vi "read_data.vi"(8 "error in (no error)":errorcluster, 10 "bytes to read":i32, 11 "MH100301DMC in":refnum<class "StageMH100301DMC.lvclass">) -> (0 "error out":errorcluster, 2 "hex data string":string, 3 "MH100301DMC out":refnum<class "StageMH100301DMC.lvclass">)   [LabVIEW 2010]
uses:
  StageMH100301DMC.lvclass
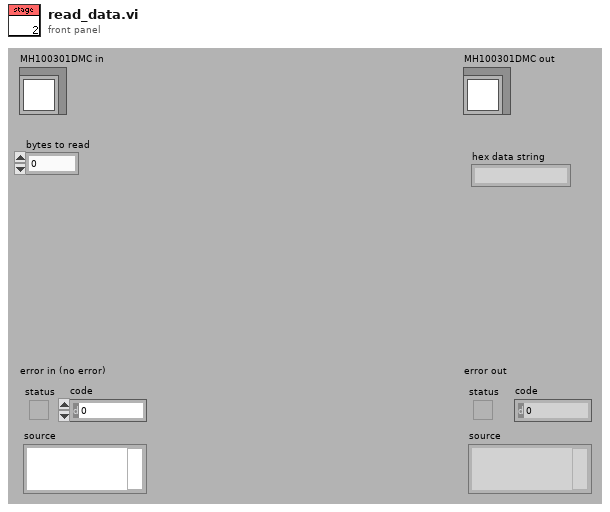
[diagram p1: front panel]
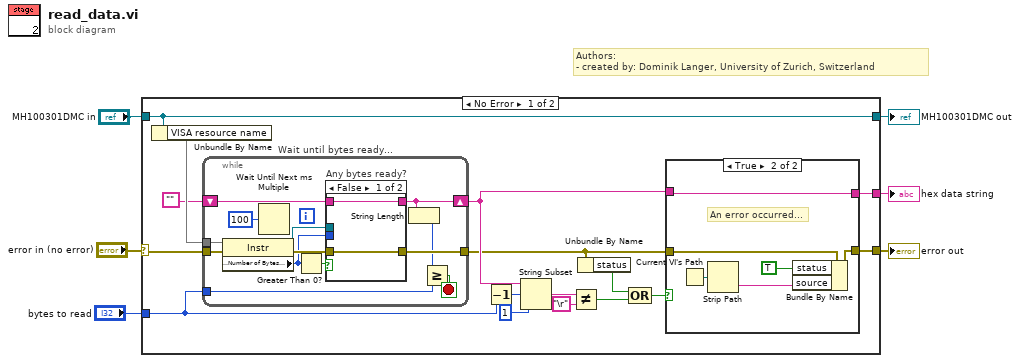
[diagram p0: block diagram]
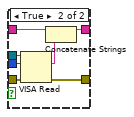
[diagram p2: hidden frame]
diagram:
  # "Authors: \n- created by: Dominik Langer, University of Zurich, Switzerland"
  n1 = case shown="No Error" "error in (no error)" {
    selector: "error in (no error)" -> [w12 w54]
    tunnel: [w18 w54] -> w6
    tunnel: [w7 w53] -> w4
    tunnel: "MH100301DMC in" -> [w7 w53]
    tunnel: [w17 _] -> w3
    tunnel: "bytes to read" -> [w8 _]
    frame No Error {
      n2 = Unbundle By Name(w7) -> ("VISA resource name"=w13)
      n3 = while "Wait until bytes ready..." {
        tunnel: w13 -> [w35]
        tunnel: w12 -> [w34]
        tunnel: [w30] -> w10
        tunnel: w8 -> [w26]
        shift-right: [w28] -> w11
        shift-left: "" -> [w29]
        stop <- w25 stop-if-true
        n4 = property class="Instr"(reference=w35, error in=w34) -> (reference out=w31:refnum<visa-resource-name>, error out=w32:errorcluster, "Serial Settings:Number of Bytes at Serial Port"=w23:u32)
        n5 = Wait Until Next ms Multiple(millisecond multiple=u32 100) -> ()  [unwired: 1 out]
        n6 = Greater Than 0?(x=w23) -> (x > 0?=w24:bool)
        n7 = case "Any bytes ready?" shown="False" w24 {
          tunnel: w32 -> [w37 w44]
          tunnel: w31 -> [_ w43]
          tunnel: [w37 w42] -> w30
          tunnel: w29 -> [w36 w41]
          tunnel: [w36 w39] -> w28
          tunnel: w23 -> [_ w38]
          frame False {
          }
          frame True {
            n8 = VISA Read(VISA resource name=w43, byte count=w38, error in (no error)=w44) -> (read buffer=w40:string, error out=w42:errorcluster)  [unwired: 2 out]
            n9 = Concatenate Strings(w41, w40) -> (w39:string)
          }
        }
        n10 = String Length(string=w28) -> (length=w27:i32)
        n11 = Greater Or Equal?(x=w27, y=w26) -> (x >= y?=w25:bool)
      }
      n12 = Decrement(x=w8) -> (x-1=w22:i32)
      n13 = String Subset(string=w11, offset (0)=w22, length (rest)=1 ("length (rest)")) -> (substring=w20:string)
      n14 = Not Equal?(x=w20, y="\r") -> (x != y?=w16:bool)
      n15 = Unbundle By Name(w10) -> ("status"=w15:bool)
      n16 = Compound Arithmetic op=OR(w15, w16) -> (w14:bool)
      n17 = case shown="True" w14 {
        tunnel: w10 -> [w46 w52]
        tunnel: [w46 w51] -> w18
        tunnel: [w45 w47] -> w17
        tunnel: w11 -> [w45 w47]
        frame False {
          # "No error..."
        }
        frame True {
          # "An error occurred..."
          n18 = Current VI's Path() -> (path=w49:path)
          n19 = Strip Path(path=w49) -> (name=w48:string)  [unwired: 1 out]
          n20 = Bundle By Name(cluster=w52, "status"=TRUE, "source"=w48) -> (w51:errorcluster)
        }
      }
    }
    frame Error {
    }
  }
  "error out" <- w6
  "MH100301DMC out" <- w4
  "hex data string" <- w3
